vi "Deque experiment.vi"(0 "object in":refnum<class "ExperimentSeries2.lvclass">, 5 "error in (no error)":errorcluster) -> (14 "object out":refnum<class "ExperimentSeries2.lvclass">, 16 "Experiment2":refnum<class "Experiment2.lvclass">, 17 "timed out?":bool, 19 "error out":errorcluster)   [LabVIEW 2021, in "ExperimentSeries2.lvclass"]
uses:
  ExperimentSeries2.lvclass
  ExperimentSeries2.lvclass/ExperimentSeries2.ctl
  Experiment2_class/Experiment2.lvclass
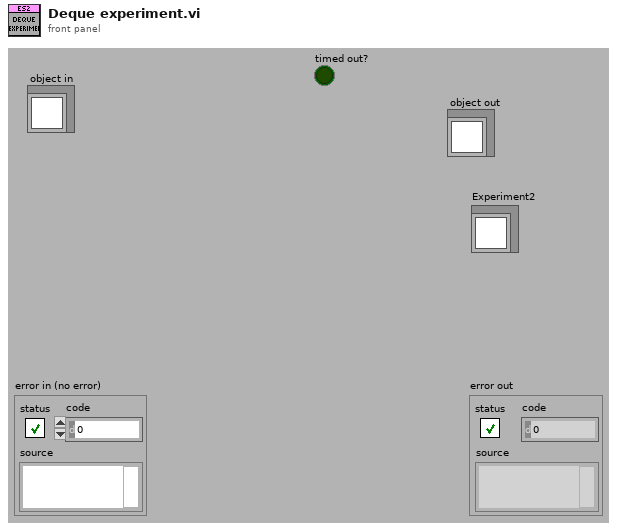
[diagram p1: front panel]
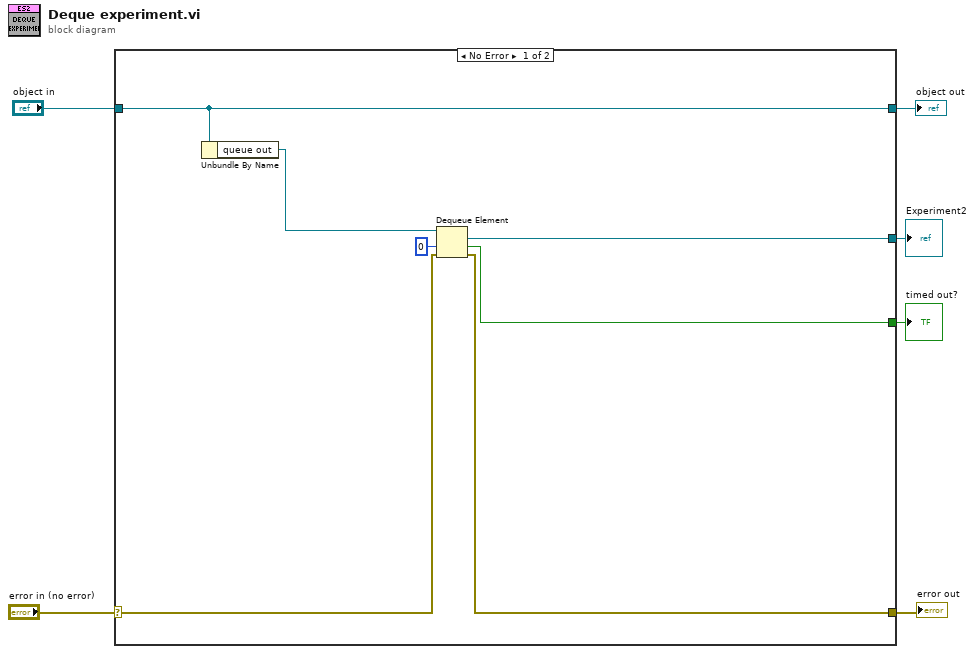
[diagram p0: block diagram]
diagram:
  n1 = case shown="No Error" "error in (no error)" {
    selector: "error in (no error)" -> [w11 w15]
    tunnel: [w10 w15] -> w5
    tunnel: [w13 w14] -> w3
    tunnel: "object in" -> [w13 w14]
    tunnel: [w9 _] -> w1
    tunnel: [w7 _] -> w2
    frame No Error {
      n2 = Unbundle By Name(w13) -> ("queue out"=w12:refnum<queue>)
      n3 = Dequeue Element(queue=w12, timeout in ms (-1)=0, error in (no error)=w11) -> (element=w9:refnum<class "Experiment2.lvclass">, timed out?=w7:bool, error out=w10:errorcluster)  [unwired: 1 out]
    }
    frame Error {
    }
  }
  "error out" <- w5
  "object out" <- w3
  "timed out?" <- w2
  "Experiment2" <- w1
